vi "#253_MAV_MSG_STATUSTEXT_ENCODE.vi"(10 "packet_sequence_in":u8, 11 "STATUSTEXT":T1={"severity"=enum."MAV_SEVERITY_INFO", "id"=0, "chunk_seq"=0, "text"="Labview Ground Control Station 0.1", "self"={"system_id"=255, "component_id"=190}}) -> (2 "packet_sequence_out":u8, 3 "mavlink_buffer_out":u8[](array[numeric]))   [LabVIEW 2023]
panel:
  out "unsigned byte array":u8[](array[numeric])
  out "string":string
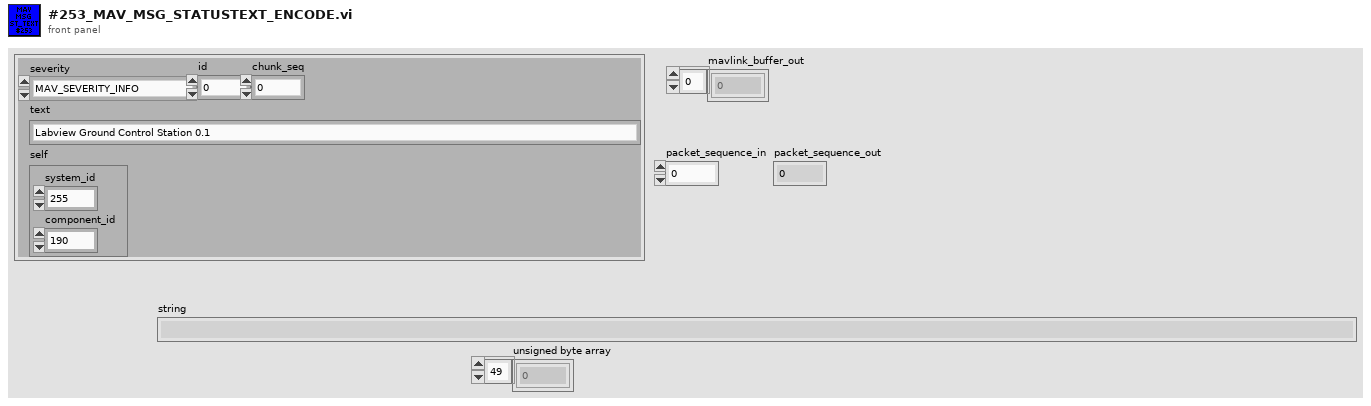
[diagram p1: front panel]
types:
  T1 = cluster{"severity":enum8{"MAV_SEVERITY_EMERGENCY", "MAV_SEVERITY_ALERT", "MAV_SEVERITY_CRITICAL", "MAV_SEVERITY_ERROR", "MAV_SEVERITY_WARNING", "MAV_SEVERITY_NOTICE", "MAV_SEVERITY_INFO", "MAV_SEVERITY_DEBUG"}, "id":u16, "chunk_seq":u8, "text":string, "self":cluster{"system_id":u8, "component_id":u8}}
  T2 = enum8{"MAV_SEVERITY_EMERGENCY", "MAV_SEVERITY_ALERT", "MAV_SEVERITY_CRITICAL", "MAV_SEVERITY_ERROR", "MAV_SEVERITY_WARNING", "MAV_SEVERITY_NOTICE", "MAV_SEVERITY_INFO", "MAV_SEVERITY_DEBUG"}
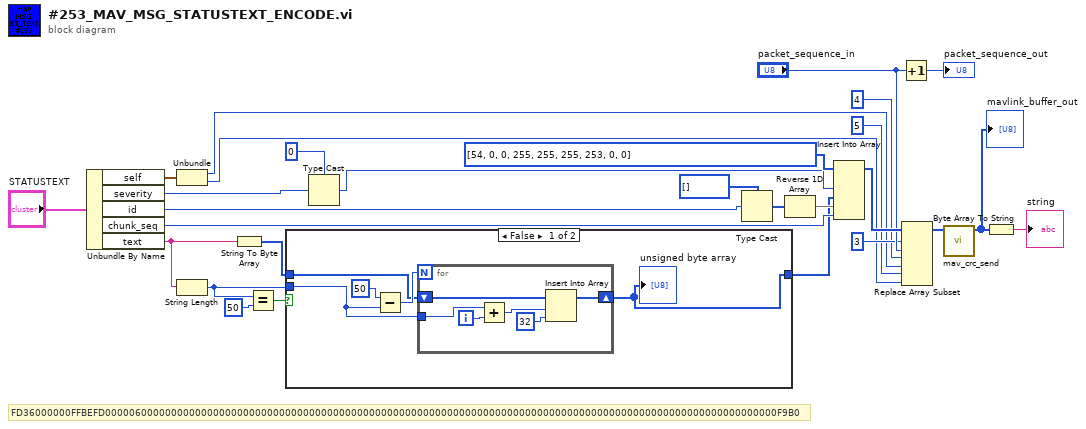
[diagram p0: block diagram]
diagram:
  # "FD36000000FFBEFD0000060000000000000000000000000000000000000000000000000000000000000000000000000000000000000000000000000000000000F9B0"
  n1 = Unbundle By Name("STATUSTEXT") -> ("self"=w24:cluster{"system_id":u8, "component_id":u8}, "severity"=w15:T2, "id"=w13:u16, "chunk_seq"=w9:u8, "text"=w5:string)
  n2 = Unbundle(w24) -> ("system_id"=w19:u8, "component_id"=w18:u8)
  n3 = String Length(string=w5) -> (length=w6:i32)
  n4 = String To Byte Array(string=w5) -> (unsigned byte array=w4:u8[])
  n5 = Equal?(x=w6, y=50) -> (x = y?=w7:bool)
  n6 = case shown="False" w7 {
    tunnel: [w30 w40] -> w1
    tunnel: w4 -> [w31 w40]
    tunnel: w6 -> [w29 _]
    frame False {
      n7 = Subtract(x=50, y=w29) -> (x-y=w32:i32)
      n8 = for {
        N: w32 -> [_]
        shift-right: [w39] -> w30
        shift-left: w31 -> [w38]
        tunnel: w29 -> [w36]
        i -> [w37]
        n9 = Add(x=w36, y=w37) -> (x+y=w35:i32)
        n10 = Insert Into Array(array=w38, index=w35, new element=u8 32 ("new element/subarray")) -> (w39:u8[])
      }
      "unsigned byte array" <- w30
    }
    frame True {
    }
  }
  n11 = Type Cast(type=u8 0 ("index"), x=w15) -> (*(type *) &x=w14:u8)
  n12 = Type Cast(type=u8[] [] ("index"), x=w13) -> (*(type *) &x=w11:u8[])
  n13 = Reverse 1D Array(array=w11) -> (reversed array=w10:u8[])
  n14 = Insert Into Array(array=u8[] [54, 0, 0, 255, 255, 255, 253, 0, 0], new element #1=w14, new element #2=w1, new element #3=w10, new element #4=w9) -> (w27:u8[])  [unwired: 1 in]
  n15 = Increment(x="packet_sequence_in") -> (x+1=→"packet_sequence_out":u8)
  n16 = Replace Array Subset(array=w27, new element #1="packet_sequence_in", index #1=3 ("index"), new element #2=w19, index #2=4 ("index"), new element #3=w18, index #3=5 ("index")) -> (w17:u8[])
  n17 = call "mav_crc_send.vi"("Byte In"=w17) -> ("Output Byte"=w3:u8[])  [unwired: 10 in]
  "mavlink_buffer_out" <- w3
  n18 = Byte Array To String(unsigned byte array=w3) -> (string=→"string":string)
